vi "daqmx_resistance.vi"() -> ()   [LabVIEW 2019]
uses:
  <vilib>/DAQmx/create/channels.llb/DAQmx Create Channel (AI-Resistance).vi
  <vilib>/DAQmx/configure/timing.llb/DAQmx Timing (Sample Clock).vi
  <vilib>/DAQmx/configure/task.llb/DAQmx Configure Logging (TDMS).vi
  <resource>/objmgr/daqmx.rc
panel:
  out "data":waveform(dbl)={"t0"=timestamp(3652936674.568203 s since 1904-01-01), "dt"=0.0025, "Y"=[346.556966635946, 346.551423770195, 346.54939734615704, 346.547966929189, 346.55321179140503, 346.55243698221403, 346.551602572316, 346.54629810939304, 346.553569395647, 346.546774915049], "attributes"=variant("NI_ChannelName"=variant(string "cDAQ1Mod1/ai0"), "NI_UnitDescription"=variant(string "Ohms"))}
  in  "NI-9217":tag="cDAQ1Mod1/ai0"
  out "Error Out":errorcluster
  in  "TDMS File":path=path "C:/Python/projects/nitdms/tests/tdms_files/daqmx_resistance.tdms"
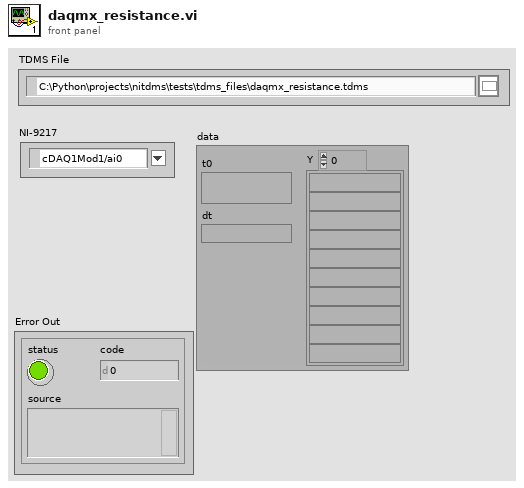
[diagram p1: front panel]
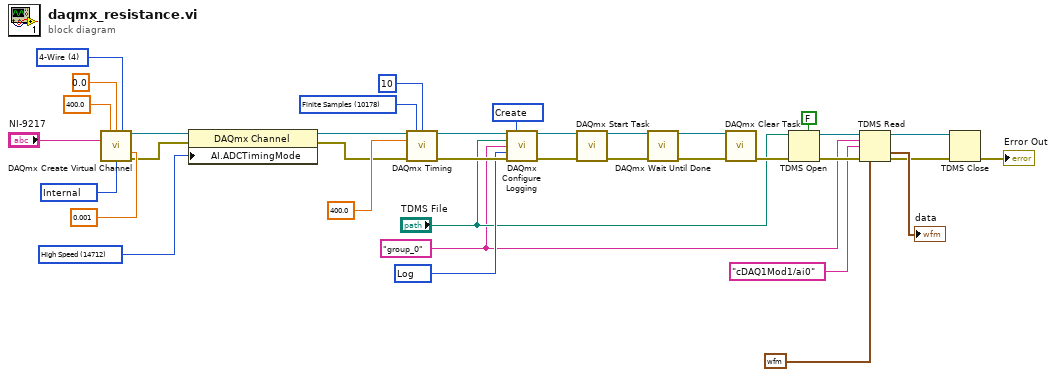
[diagram p0: block diagram]
diagram:
  w3 = 14712 items=["Automatic"=16097, "High Resolution"=10195, "High Speed"=14712, "Best 50 Hz Rejection"=14713, "Best 60 Hz Rejection"=14714, "Custom"=10137] ("AI.ADCTimingMode")
  w7 = 10200 items=["Internal"=10200, "External"=10167, "None"=10230] ("current excitation source")
  w8 = 4 items=["2-Wire"=2, "3-Wire"=3, "4-Wire"=4] ("resistance configuration")
  w29 = 10178 items=["Finite Samples"=10178, "Continuous Samples"=10123, "Hardware Timed Single Point"=12522] ("sample mode")
  w32 = 15844 items=["Off"=10231, "Log"=15844, "Log and Read"=15842] ("logging mode")
  w18 = "group_0" ("group name")
  w33 = 15848 items=["Open"=10437, "Open or Create"=15846, "Create or Replace"=15847, "Create"=15848] ("operation")
  n1 = call-poly <vilib>:"DAQmx Create Virtual Channel.vi"("maximum value"=400.0, "minimum value"=0.0, "resistance configuration"=w8, "physical channels"="NI-9217", "current excitation value"=0.001, "current excitation source"=w7) -> ("task out"=w5:refnum<k21>, "error out"=w4:errorcluster)  [unwired: 8 in]
  n2 = property class="DAQmx Channel"(reference=w5, error in=w4, "AI.ADCTimingMode"=w3) -> (reference out=w1:refnum<k21>, error out=w2:errorcluster)
  n3 = call-poly <vilib>:"DAQmx Timing.vi"("task/channels in"=w1, "sample mode"=w29, "samples per channel"=10, "rate"=400.0, "error in"=w2) -> ("task out"=w34:refnum<k21>, "error out"=w35:errorcluster)  [unwired: 9 in]
  n4 = call-poly <vilib>:"DAQmx Configure Logging.vi"("task/channels in"=w34, "operation"=w33, "file path"="TDMS File", "group name"=w18, "logging mode"=w32, "error in"=w35) -> ("task out"=w30:refnum<k21>, "error out"=w31:errorcluster)  [unwired: 8 in]
  n5 = call <vilib>:"DAQmx Start Task.vi"("task/channels in"=w30, "error in"=w31) -> ("task out"=w26:refnum<k21>, "error out"=w27:errorcluster)  [unwired: 12 in]
  n6 = call <vilib>:"DAQmx Wait Until Done.vi"("task/channels in"=w26, "error in"=w27) -> ("task out"=w24:refnum<k21>, "error out"=w25:errorcluster)  [unwired: 12 in]
  n7 = call <vilib>:"DAQmx Clear Task.vi"("task in"=w24, "error in"=w25) -> ("error out"=w23:errorcluster)  [unwired: 13 in]
  n8 = TDMS Open(5:FALSE ("create index file? (T)"), 8:w23, 11:"TDMS File") -> (0:w20:errorcluster, 3:w19:refnum<k34>)  [unwired: 4 in]
  n9 = TDMS Read(0:w19, 5:w18, 7:"cDAQ1Mod1/ai0" ("channel name(s) in"), 11:w20, 12:waveform(dbl) {"t0"=timestamp(0 s since 1904-01-01), "dt"=1.0, "Y"=[]} ("Waveform")) -> (4:w12:refnum<k34>, 10:→"data":waveform(dbl), 15:w13:errorcluster)  [unwired: 3 in, 3 out]
  n10 = TDMS Close(8:w13, 11:w12) -> (0:→"Error Out":errorcluster)  [unwired: 1 out]
